vi "FTW-Test-JSON-Deserialize.vi"() -> (0 "Test Result":errorcluster)   [LabVIEW 2018]
uses:
  663dc49e-eb3d-48d2-a836-78c41eeedf52.vi
  9ca8cdbe-7837-4bea-822a-2d858f5714f1.vi
  22b0dbe8-973d-4a85-a26b-d5ee9b26b942.vi
  f1517575-305e-48fc-953f-4c22cb25f4e8.vi
panel:
  out "JSON String (UTF-8)":string
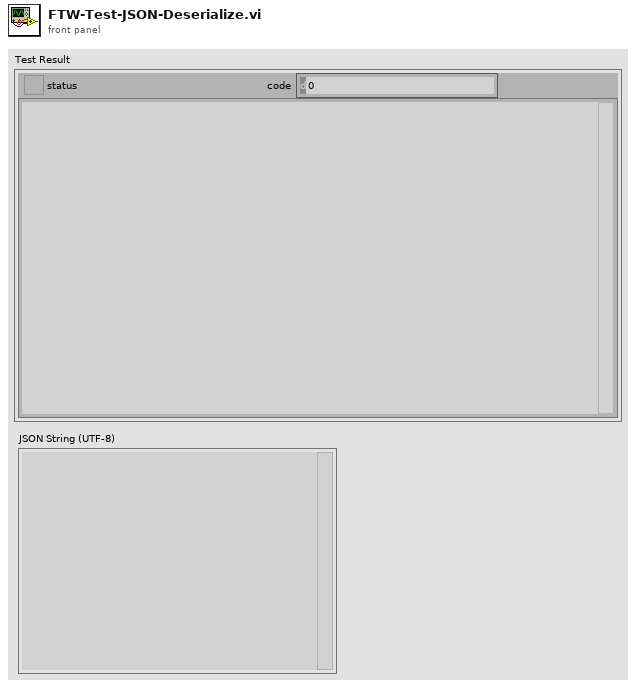
[diagram p1: front panel]
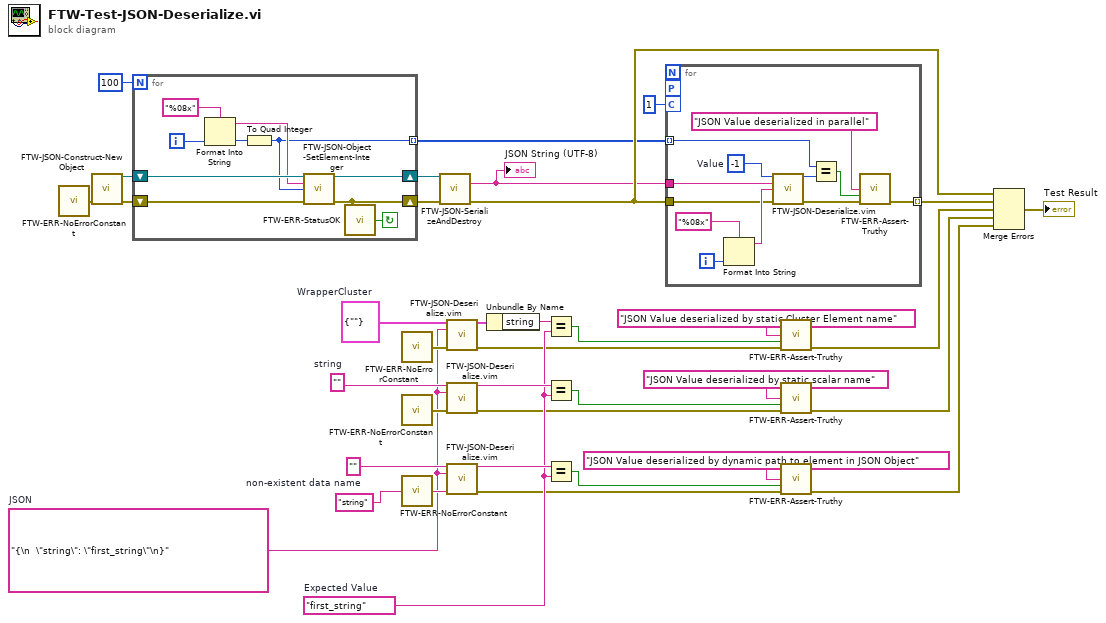
[diagram p0: block diagram]
diagram:
  w19 = ""  # non-existent data name
  w27 = ""  # string
  w20 = "first_string"  # Expected Value
  w18 = "{\n  \"string\": \"first_string\"\n}"  # JSON
  w29 = cluster{"string":string} {"string"=""}  # WrapperCluster
  n1 = call "FTW-ERR-NoErrorConstant.vi"() -> ("no error"=w35:errorcluster)
  n2 = call "FTW-JSON-Construct-NewObject.vi"("error in"=w35) -> ("JSON"=w34:refnum<class "FTW-Container.lvclass">, "error out"=w33:errorcluster)  [unwired: 13 in]
  n3 = for {
    N: 100 -> [_]
    shift-right: [w39] -> w15
    shift-left: w33 -> [w43]
    shift-right: [w44] -> w16
    shift-left: w34 -> [w45]
    tunnel: [w37] -> w17 mode=indexing
    i -> [w42]
    stop <- w38 continue-if-true
    n4 = Format Into String(format string="%08x", w42) -> (resulting string=w41:string)  [unwired: 2 in, 1 out]
    n5 = To Quad Integer(1:w42) -> (0:w37:i64)
    n6 = call "FTW-JSON-Object-SetElement-Integer.vi"("JSON"=w45, "Key"=w41, "Value"=w37, "error in"=w43) -> ("JSON out"=w44:refnum<class "FTW-Container.lvclass">, "error out"=w39:errorcluster)  [unwired: 10 in]
    n7 = call "FTW-ERR-StatusOK.vi"("error to check"=w39) -> ("Status OK?"=w38:bool)
  }
  n8 = call "FTW-ERR-NoErrorConstant.vi"() -> ("no error"=w26:errorcluster)
  n9 = call "FTW-ERR-NoErrorConstant.vi"() -> ("no error"=w25:errorcluster)
  n10 = call "FTW-ERR-NoErrorConstant.vi"() -> ()  [unwired: 1 out]
  n11 = call "FTW-JSON-SerializeAndDestroy.vi"("JSON"=w16, "error in"=w15) -> ("JSON String (UTF-8)"=w14:string, "error out"=w31:errorcluster)  [unwired: 12 in]
  "JSON String (UTF-8)" <- w14
  n12 = call "FTW-JSON-Deserialize.vim"("Type In"=w29, "JSON String"=w18, "error in"=w26) -> ("Type Out"=w28:cluster{"string":string}, "error out"=w6:errorcluster)  [unwired: 11 in]
  n13 = call "FTW-JSON-Deserialize.vim"("Type In"=w27, "JSON String"=w18, "error in"=w25) -> ("Type Out"=w23:string, "error out"=w9:errorcluster)  [unwired: 11 in]
  n14 = call "FTW-JSON-Deserialize.vim"("Type In"=w19, "JSON String"=w18, "error in"="string" ("Element Path")) -> ("Type Out"=w21:string, "error out"=w13:errorcluster)  [unwired: 11 in]
  n15 = Unbundle By Name(w28) -> ("string"=w24:string)
  n16 = Equal?(x=w24, y=w20) -> (x = y?=w7:bool)
  n17 = Equal?(x=w23, y=w20) -> (x = y?=w10:bool)
  n18 = Equal?(x=w21, y=w20) -> (x = y?=w11:bool)
  n19 = for {
    workers-P: _ -> [_]
    chunk-C: 1 -> [_]
    tunnel: w14 -> [w57]
    tunnel: [w47] -> w32 mode=indexing
    tunnel: w31 -> [w53]
    tunnel: w17 -> [w52] mode=indexing
    i -> [w55]
    w51 = i64 -1  # Value
    n20 = Format Into String(format string="%08x", w55) -> (resulting string=w56:string)  [unwired: 2 in, 1 out]
    n21 = call "FTW-JSON-Deserialize.vim"("Type In"=w51, "JSON String"=w57, 7:w56, "error in"=w53) -> ("Type Out"=w50:i64, "error out"=w48:errorcluster)  [unwired: 10 in]
    n22 = Equal?(x=w52, y=w50) -> (x = y?=w49:bool)
    n23 = call "FTW-ERR-Assert-Truthy.vi"("Assertion"="JSON Value deserialized in parallel", "Assertion holds true?"=w49, "error in"=w48) -> ("error out"=w47:errorcluster)  [unwired: 12 in]
  }
  n24 = call "FTW-ERR-Assert-Truthy.vi"("Assertion"="JSON Value deserialized by static Cluster Element name", "Assertion holds true?"=w7, "error in"=w6) -> ("error out"=w5:errorcluster)  [unwired: 12 in]
  n25 = call "FTW-ERR-Assert-Truthy.vi"("Assertion"="JSON Value deserialized by static scalar name", "Assertion holds true?"=w10, "error in"=w9) -> ("error out"=w8:errorcluster)  [unwired: 12 in]
  n26 = call "FTW-ERR-Assert-Truthy.vi"("Assertion"="JSON Value deserialized by dynamic path to element in JSON Object", "Assertion holds true?"=w11, "error in"=w13) -> ("error out"=w12:errorcluster)  [unwired: 12 in]
  n27 = Merge Errors(w31, w32, w5, w8, w12) -> (→"Test Result":errorcluster)
